vi "PH_Connection.get IP Address.vi"(2 "IP Name":string) -> (14 "1st # of IP":u8, 15 "2nd # of IP":u8, 16 "3rd # of IP":u8, 17 "4th # of IP":u8, 18 "Client found":bool, 19 "IP Address":string)   [LabVIEW 2014, in "PH_Common.lvlib"]
doc: "This VI gets the IP of an incoming IP address; IP Name might be\n\nphpc061, or phpc061.gsi.de, 140.181.17.8; output is the first to the 4th Number of the IP, the information, whether the client has been found, and the IP Address as string (140.181.xxx,yyy)."
uses:
  PH_Common.lvlib
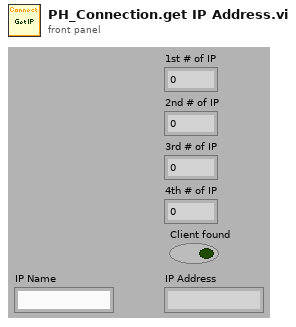
[diagram p1: front panel]
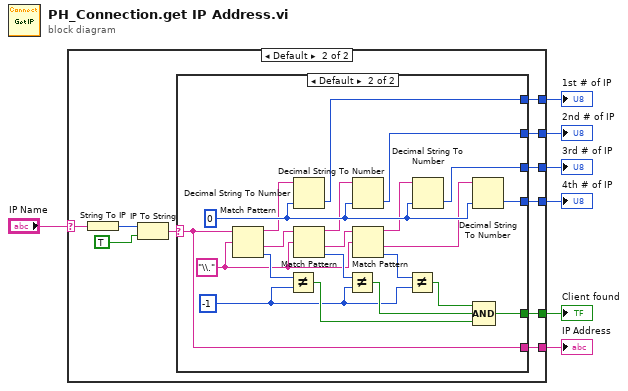
[diagram p0: block diagram]
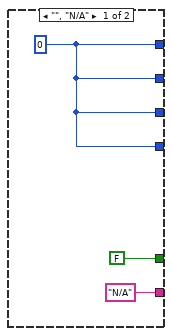
[diagram p2: hidden frame]
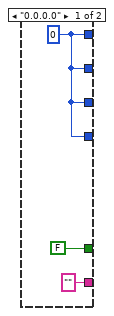
[diagram p3: hidden frame]
diagram:
  n1 = case shown="Default" "IP Name" {
    selector: "IP Name" -> [_ w14]
    tunnel: [w10 w20] -> w7
    tunnel: [w10 w19] -> w6
    tunnel: [w10 w18] -> w5
    tunnel: [w10 w17] -> w4
    tunnel: [FALSE w16] -> w3
    tunnel: ["N/A" ("name") w12] -> w2
    frame "", "N/A" {
      w10 = u8 0
    }
    frame Default {
      n2 = String To IP(1:w14) -> (0:w15:u32)
      n3 = IP To String(1:TRUE ("dot notation? (F)"), 2:w15) -> (0:w13:string)
      n4 = case shown="Default" w13 {
        selector: w13 -> [_ w24]
        tunnel: [w21 w44] -> w20
        tunnel: [w21 w43] -> w19
        tunnel: [w21 w42] -> w18
        tunnel: [w21 w41] -> w17
        tunnel: [FALSE w40] -> w16
        tunnel: ["" w24] -> w12
        frame "0.0.0.0" {
          w21 = u8 0
        }
        frame Default {
          w36 = -1 ("y")
          w32 = u8 0 ("default (0 I32)")
          w27 = "\\." ("regular expression")
          n5 = Match Pattern(string=w24, regular expression=w27) -> (before substring=w28:string, after substring=w25:string, offset past match=w33:i32)  [unwired: 1 in, 1 out]
          n6 = Not Equal?(x=w33, y=w36) -> (x != y?=w39:bool)
          n7 = Decimal String To Number(string=w28, default (0L)=w32) -> (number=w44:u8)  [unwired: 1 in, 1 out]
          n8 = Match Pattern(string=w25, regular expression=w27) -> (before substring=w29:string, after substring=w26:string, offset past match=w35:i32)  [unwired: 1 in, 1 out]
          n9 = Not Equal?(x=w35, y=w36) -> (x != y?=w38:bool)
          n10 = Decimal String To Number(string=w29, default (0L)=w32) -> (number=w43:u8)  [unwired: 1 in, 1 out]
          n11 = Match Pattern(string=w26, regular expression=w27) -> (before substring=w30:string, after substring=w31:string, offset past match=w34:i32)  [unwired: 1 in, 1 out]
          n12 = Not Equal?(x=w34, y=w36) -> (x != y?=w37:bool)
          n13 = Decimal String To Number(string=w30, default (0L)=w32) -> (number=w42:u8)  [unwired: 1 in, 1 out]
          n14 = Decimal String To Number(string=w31, default (0L)=w32) -> (number=w41:u8)  [unwired: 1 in, 1 out]
          n15 = Compound Arithmetic op=AND(w37, w38, w39) -> (w40:bool)
        }
      }
    }
  }
  "1st # of IP" <- w7
  "2nd # of IP" <- w6
  "3rd # of IP" <- w5
  "4th # of IP" <- w4
  "Client found" <- w3
  "IP Address" <- w2
